vi "Parse Response.vi"(8 "error in (no error)":errorcluster, 10 "Data":u64) -> (0 "error out":errorcluster, 1 "Data 3":u16, 2 "Data 2":u16, 3 "Data 1":u16, 4 "Command":u8, 5 "Target ID":u8)   [LabVIEW 2020, in "BCI-1553 API.lvlib" / "FPGA Interface.lvlib" / "FPGA Interface.lvclass"]
doc: "Parses response data from a component in the 1553 Session."
uses:
  FPGA Interface.lvclass
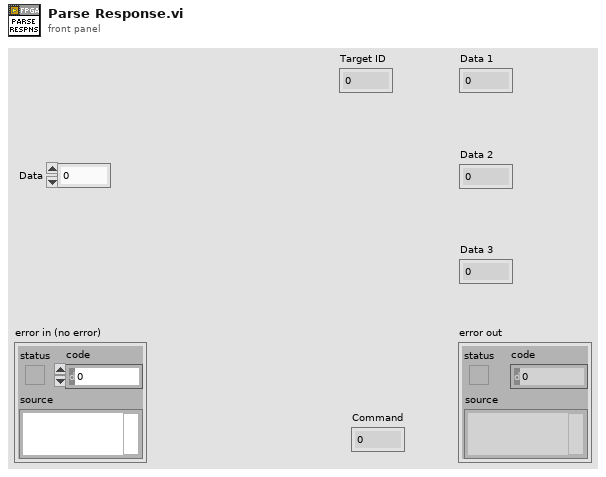
[diagram p1: front panel]
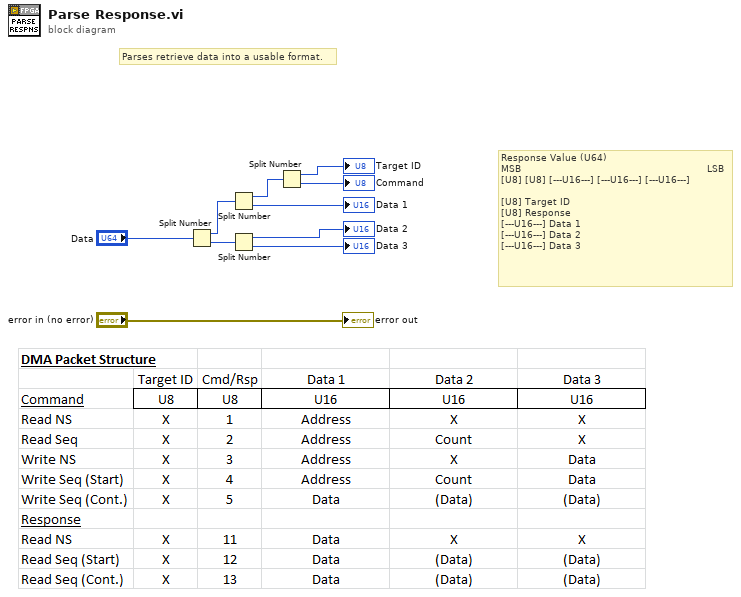
[diagram p0: block diagram]
diagram:
  # "Response Value (U64)\nMSB                                                              LSB\n[U8] [U8] [---U16---] [---U16---] [---U16---]\n\n[U8] Target ID\n[U8] Response\n[---U16---] Data 1\n[---U16---] Data 2\n[---U16---] Data 3"
  # "Parses retrieve data into a usable format."
  n1 = Split Number(x="Data") -> (hi(x)=w1:u32, lo(x)=w3:u32)
  n2 = Split Number(x=w1) -> (hi(x)=w2:u16, lo(x)=→"Data 1":u16)
  n3 = Split Number(x=w3) -> (hi(x)=→"Data 2":u16, lo(x)=→"Data 3":u16)
  n4 = Split Number(x=w2) -> (hi(x)=→"Target ID":u8, lo(x)=→"Command":u8)
  "error out" <- "error in (no error)"
